vi "Search Events.vi"(7 "Action (Get)":enum16{"Initialize", "Get", "Destroy"}(ring)=enum."Get", 8 "error in":errorcluster) -> (0 "error out":errorcluster, 3 "SearchEvents":T1)   [LabVIEW 2013, in "LVTM.lvlib"]
uses:
  LVTM.lvlib
  Controls_LVTM/SearchEvents.ctl
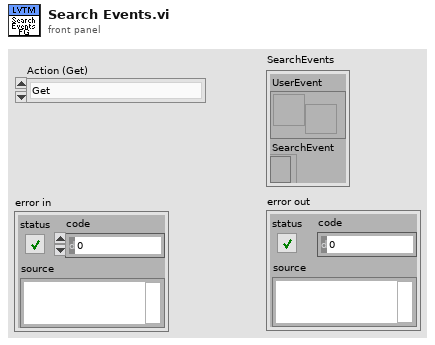
[diagram p1: front panel]
types:
  T1 = typedef "LVTM.lvlib/SearchEvents.ctl" = cluster{"UserEvent":refnum<user-event>, "SearchEvent":refnum<event-registration>}
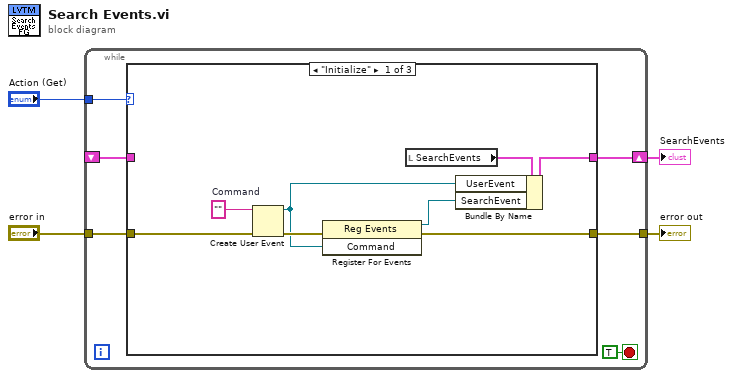
[diagram p0: block diagram]
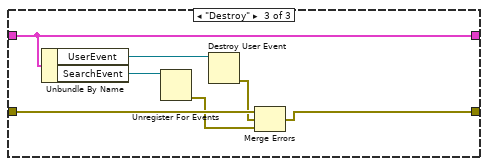
[diagram p3: hidden frame]
diagram:
  n1 = while {
    tunnel: "Action (Get)" -> [w10]
    shift-right: [w7] -> w1
    shift-left: _ -> [w6]
    tunnel: "error in" -> [w9]
    tunnel: [w8] -> w2
    stop <- TRUE stop-if-true
    n2 = case shown="\"Initialize\"" w10 {
      tunnel: w9 -> [w17 w19 w27]
      tunnel: [w15 w19 w26] -> w8
      tunnel: [w12 w20 w24] -> w7
      tunnel: w6 -> [_ w20 w24]
      frame "Initialize" {
        w18 = ""  # Command
        n3 = Create User Event(user event datatype=w18, error in=w17) -> (user event=w14:refnum<user-event>, error out=w16:errorcluster)
        n4 = register-events(error in=w16, w14) -> (reference out=w13:refnum<event-registration>, error out=w15:errorcluster)  [unwired: 1 in]
        n5 = local read "SearchEvents"() -> (w11:T1)
        n6 = Bundle By Name(cluster=w11, "UserEvent"=w14, "SearchEvent"=w13) -> (w12:T1)
      }
      frame "Get" {
      }
      frame "Destroy" {
        n7 = Unbundle By Name(w24) -> ("UserEvent"=w23:refnum<user-event>, "SearchEvent"=w22:refnum<event-registration>)
        n8 = Unregister For Events(event registration refnum=w22) -> (error out=w21:errorcluster)  [unwired: 1 in]
        n9 = Destroy User Event(user event=w23) -> (error out=w25:errorcluster)  [unwired: 1 in]
        n10 = Merge Errors(w27, w25, w21) -> (w26:errorcluster)
      }
    }
  }
  "error out" <- w2
  "SearchEvents" <- w1
